vi "XY - Graph As Chart Demo.vi"() -> ()   [LabVIEW 2012]
uses:
  <vilib>/ptbypt/NI_PtbyPt.lvlib
panel:
  out "XY Graph":cluster{dbl[], dbl[]}(graph)
  in  "Chart History":i32=500 caption="Maximum Number of Data Points (Chart History)"
  in  "stop":bool
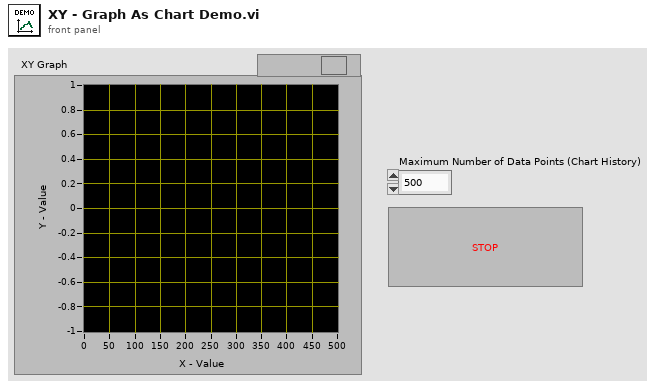
[diagram p1: front panel]
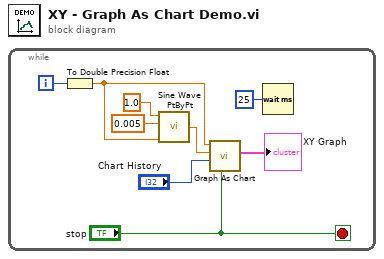
[diagram p0: block diagram]
diagram:
  n1 = while {
    i -> [w3]
    stop <- "stop" stop-if-true
    n2 = To Double Precision Float(number=w3) -> (double precision float=w2:dbl)
    n3 = call <vilib>:"Sine Wave PtByPt.vi"("time"=w2, "frequency"=0.005, "amplitude"=1.0) -> ("sine wave"=w4:dbl)  [unwired: 1 in]
    n4 = call "Graph As Chart.vi"("Clear Graph?"="stop", "Chart History (10,000)"="Chart History", "Y Value"=w4, "X Value"=w2) -> ("XY Graph"=→"XY Graph":cluster{dbl[], dbl[]})  [unwired: 7 in]
    n5 = Wait (ms)(milliseconds to wait=u32 25) -> ()  [unwired: 1 out]
  }
